vi "Find host address.vi"(0 "System number":i32=1 min=1 step=1, 1 "Port":i32=50000, 2 "Controller names":string[](array[string]), 3 "Mode":T1(ring), 5 "error in":errorcluster, 12 "Stop refnum":refnum<vi>) -> (14 "Address":string[](array[string]), 15 "ID":string[](array[string]), 16 "All Addresses":string[](array[string]), 17 "All IDs":string[](array[string]), 19 "error out":errorcluster)   [LabVIEW 2020]
doc: "Performs an UDP broadcast and returns IP addresses of all controllers matching Controller name. VI will also stop if Stop refnum or Local stop is TRUE.\n\nC-413: Controller names = C-413, Mode = Find XPort by UDP, Port = 30718\nC-413: Controller names = C-413, Mode = Find USR-K3 by UDP, Port = 1901\nC-702: Controller names = C-702, Mode = Find controller by UDP, Port = 50000\nC-867: Controller names = C-867, Mode = Find controller by UDP, Port = 50000\nC-884: Controller names = C-884, Mode = Find controller by UDP, Port = 50000\nC-885: Controller names = C-885, Mode = Find controller by UDP, Port = 50000\nC-886: Controller names = C-886, Mode = Find controller by UDP, Port = 50000\nC-891: Controller names = C-891, Mode = Find XPort by UDP, Port = 30718\nE-135: Controller names = E-135, Mode = Find USR-K3 by UDP, Port = 1901\nE-517: Controller names = E-517, Mode = Find controller by UDP, Port = 50000\nE-518: Controller names = E-518, Mode = Find controller by UDP, Port = 50000\nE-712: Controller names = E-712, Mode = Find controller by UDP, Port = 50000\nE-725: Controller names = E-725, Mode = Find XPort by UDP, Port = 30718\nE-727: Controller names = E-727, Mode = Find controller by UDP, Port = 50000\nE-753: Controller names = E-753, Mode = Find controller by UDP, Port = 50000\nE-754: Controller names = E-754, Mode = Find controller by UDP, Port = 50000\nE-871: Controller names = E-871, Mode = Find XPort by UDP, Port = 30718\nE-872: Controller names = E-872, Mode = Find controller by UDP, Port = 50000\nE-873: Controller names = E-873, Mode = Find XPort by UDP, Port = 30718\nE-874: Controller names = E-874, Mode = Find USR-K3 by UDP, Port = 1901\nF-206: Controller names = F-206, F-HEX, Mode = Find XPort by UDP, Port = 30718\nC-887, M-8X0: Controller names = M-8X0, HEXAPOD, Mode = Find XPort by UDP, Port = 30718"
uses:
  ProgramData/PI/LabVIEW/Low Level/Communication.llb/Available interfaces.ctl
  ProgramData/PI/LabVIEW/Low Level/Communication.llb/Global1.vi
  <vilib>/regexp/Match Regular Expression.xnode
panel:
  in  "stop":bool
  # "Performs an UDP broadcast and returns IP addresses of all controllers matching \"Controller name\"."
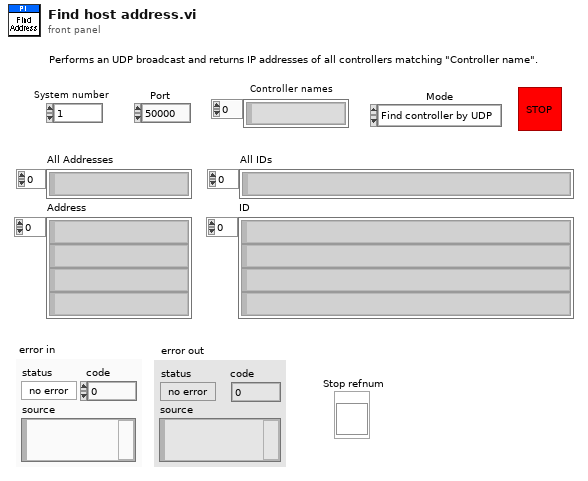
[diagram p1: front panel]
types:
  T1 = enum16{"Find controller by UDP", "Find XPort by UDP", "Find USR-K3 by UDP"}
  T2 = cluster{"Host address/name":string, "Port":i32, "Board":i32}
  T3 = typedef "Available interfaces.ctl" = u16
  T4 = cluster{"RS232 Portnumber":i32, "Timeout":i32, "RS232 Baud rate":u32, "Interface":T3, "GPIB Bus":i32, "GPIB Address":i32, "GPIB Mode":i32}
  T5 = cluster{"second":i32, "minute":i32, "hour":i32, "day of month":i32, "month":i32, "year":i32, "day of week":i32, "day of year":i32, "is DST":i32}
  T6 = cluster{"[0]":u8, "[1]":u8, "[2]":u8, "[3]":u8, "[4]":u8, "[5]":u8, "[6]":u8, "[7]":u8, "[8]":u8, "[9]":u8, "[10]":u8, "[11]":u8, "[12]":u8, "[13]":u8, "[14]":u8, "[15]":u8, "[16]":u8, "[17]":u8, "[18]":u8, "[19]":u8, "[20]":u8, "[21]":u8, "[22]":u8, "[23]":u8, "[24]":u8, "[25]":u8, "[26]":u8, "[27]":u8, "[28]":u8, "[29]":u8, "[30]":u8, "[31]":u8, "[32]":u8, "[33]":u8, "[34]":u8, "[35]":u8, "[36]":u8, "[37]":u8, "[38]":u8, "[39]":u8, "[40]":u8, "[41]":u8, "[42]":u8, "[43]":u8, "[44]":u8, "[45]":u8, "[46]":u8, "[47]":u8, "[48]":u8, "[49]":u8, "[50]":u8, "[51]":u8, "[52]":u8, "[53]":u8, "[54]":u8, "[55]":u8, "[56]":u8, "[57]":u8, "[58]":u8, "[59]":u8, "[60]":u8, "[61]":u8, "[62]":u8, "[63]":u8, "[64]":u8, "[65]":u8, "[66]":u8, "[67]":u8, "[68]":u8, "[69]":u8, "[70]":u8, "[71]":u8, "[72]":u8, "[73]":u8, "[74]":u8, "[75]":u8, "[76]":u8, "[77]":u8, "[78]":u8, "[79]":u8, "[80]":u8, "[81]":u8, "[82]":u8, "[83]":u8, "[84]":u8, "[85]":u8, "[86]":u8, "[87]":u8, "[88]":u8, "[89]":u8, "[90]":u8, "[91]":u8, "[92]":u8, "[93]":u8, "[94]":u8, "[95]":u8, "[96]":u8, "[97]":u8, "[98]":u8, "[99]":u8, "[100]":u8, "[101]":u8, "[102]":u8, "[103]":u8, "[104]":u8, "[105]":u8, "[106]":u8, "[107]":u8, "[108]":u8, "[109]":u8, "[110]":u8, "[111]":u8, "[112]":u8, "[113]":u8, "[114]":u8, "[115]":u8, "[116]":u8, "[117]":u8, "[118]":u8, "[119]":u8, "[120]":u8, "[121]":u8, "[122]":u8, "[123]":u8}
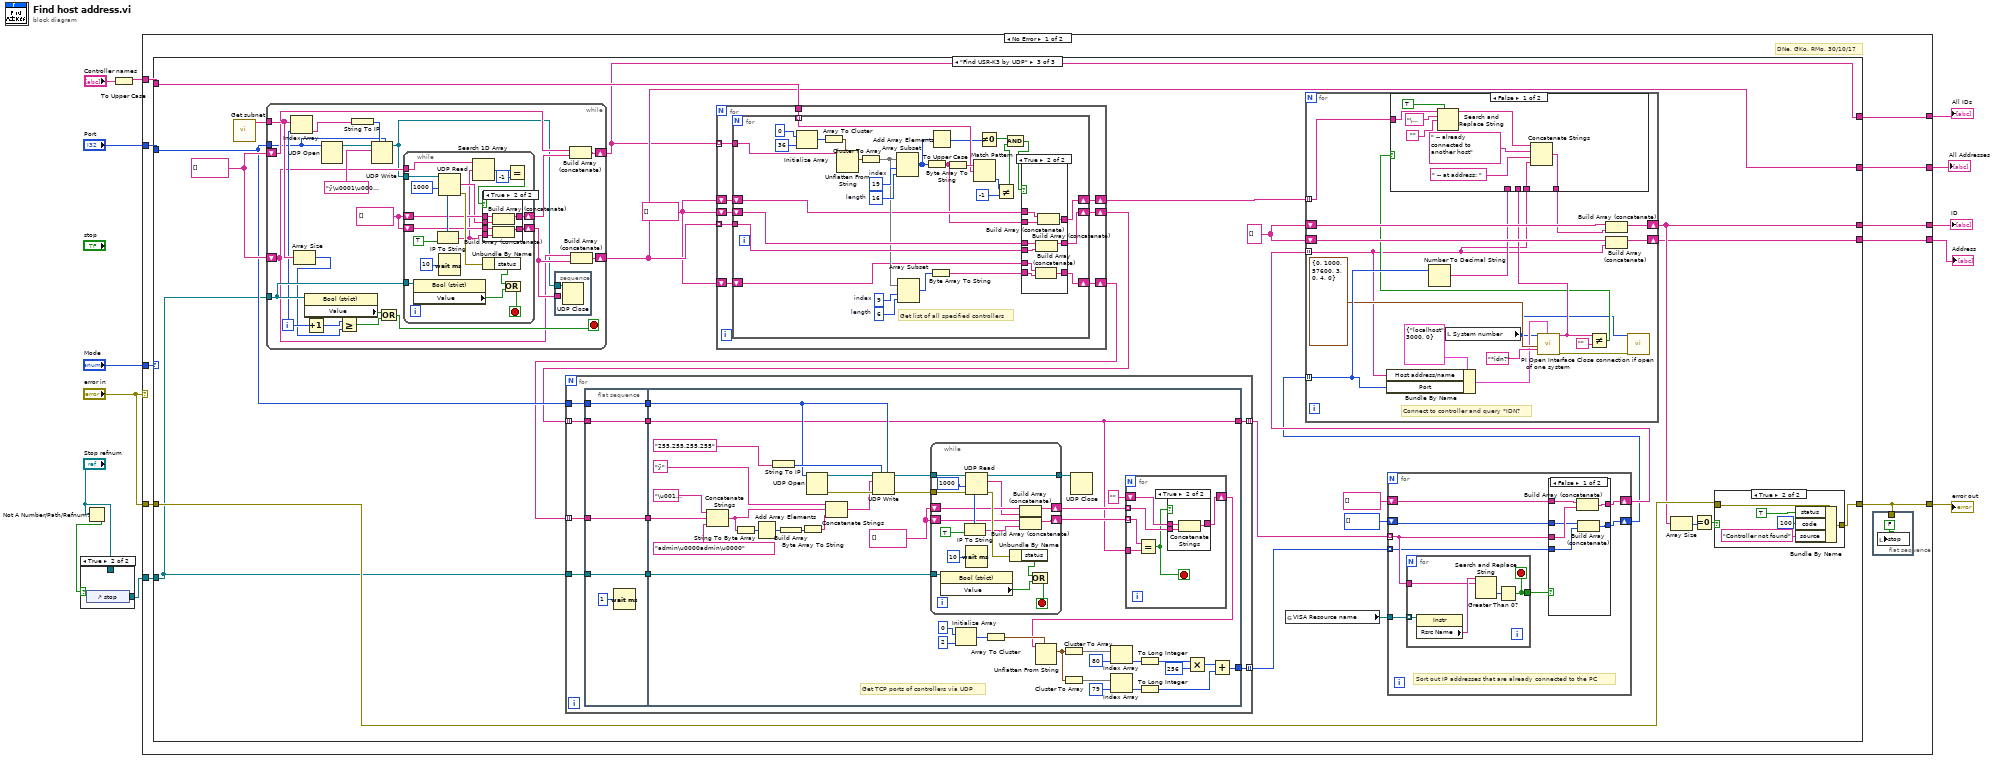
[diagram p0: block diagram]
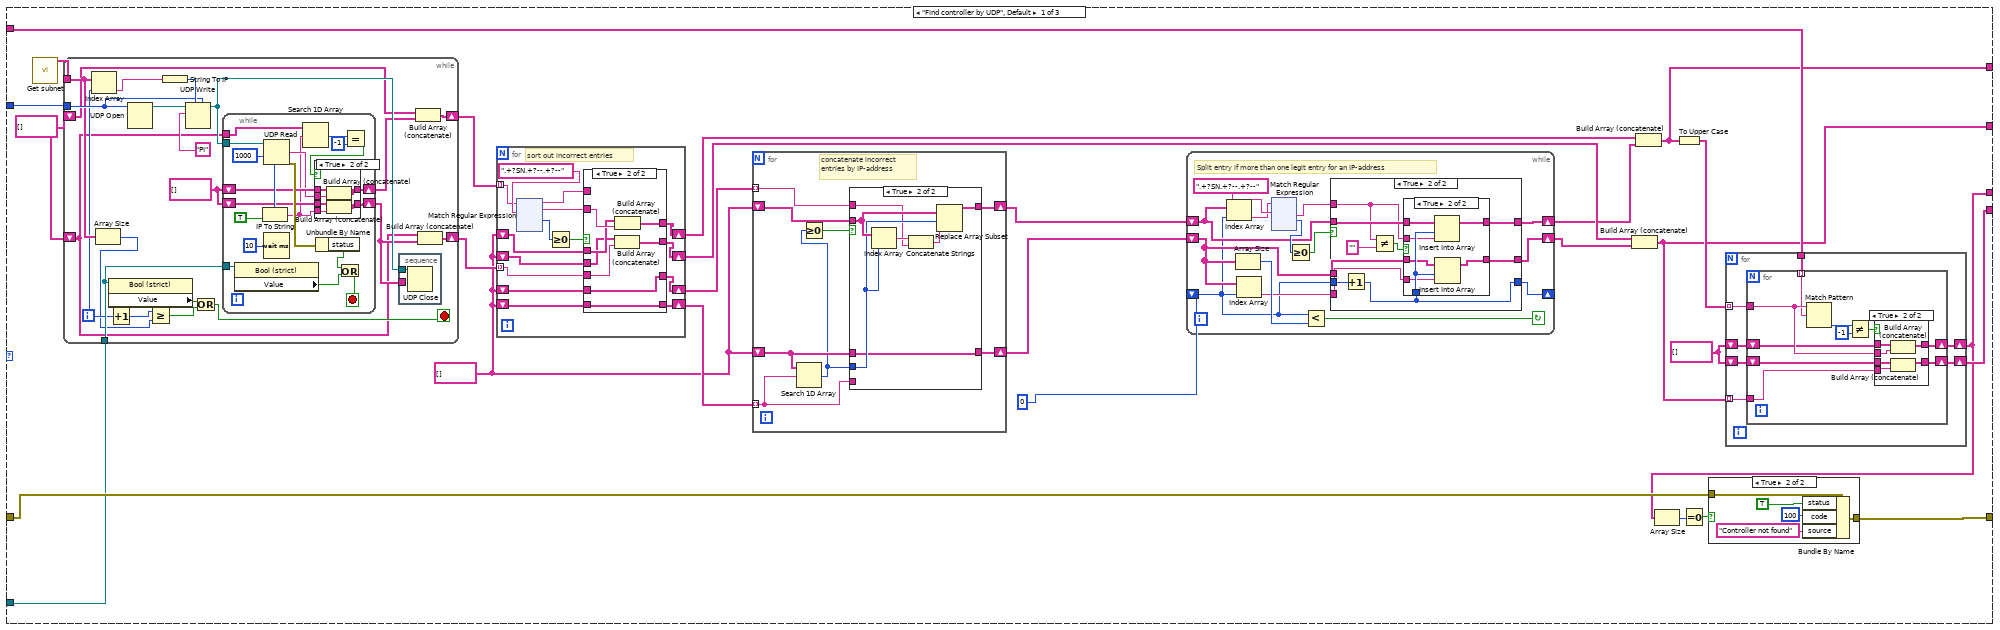
[diagram p3: hidden frame]
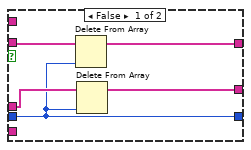
[diagram p4: hidden frame]
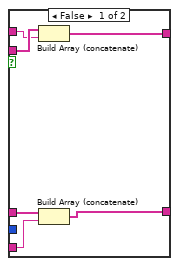
[diagram p6: hidden frame]
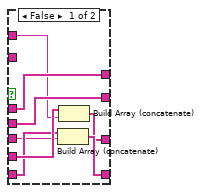
[diagram p7: hidden frame]
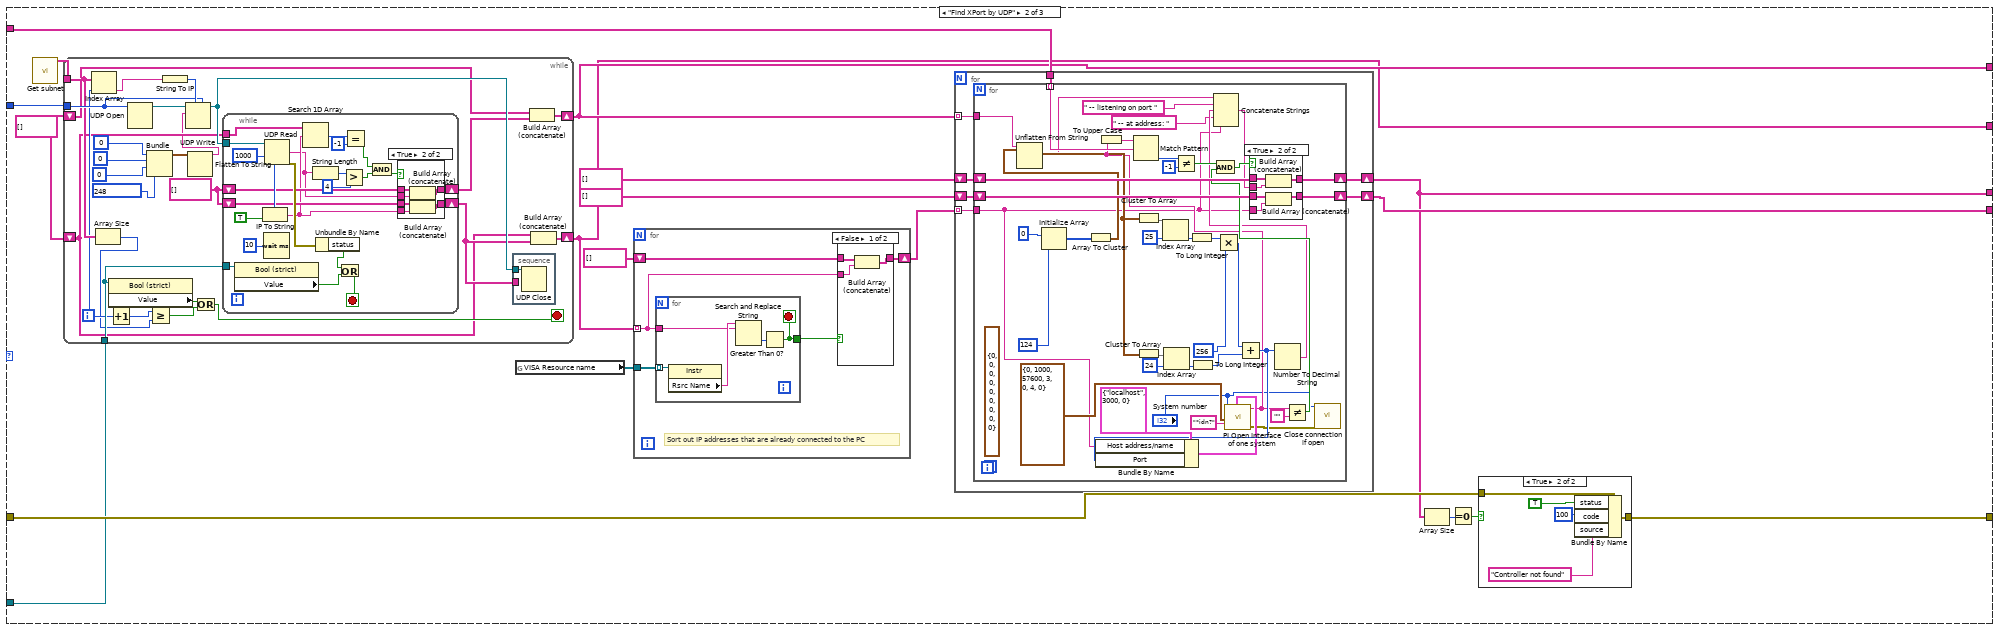
[diagram p11: hidden frame]
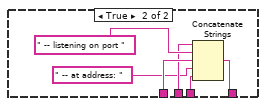
[diagram p17: hidden frame]
diagram:
  n1 = Not A Number/Path/Refnum?(number/path/refnum="Stop refnum") -> (NaN/Path/Refnum?=w7:bool)
  n2 = case shown="True" w7 {
    tunnel: [w14 w15] -> w5
    tunnel: "Stop refnum" -> [w14 _]
    frame False {
    }
    frame True {
      n3 = control-ref of="stop"() -> (w15:refnum<vi>)
    }
  }
  n4 = To Upper Case(1:"Controller names") -> (0:w4:string[])
  n5 = case shown="No Error" "error in" {
    tunnel: [w19 w880] -> w13
    tunnel: "error in" -> [w25 w880]
    tunnel: "Port" -> [w24 _]
    tunnel: "Mode" -> [w23 _]
    tunnel: w4 -> [w22 _]
    tunnel: [w21 string[] []] -> w2
    tunnel: [w17 string[] []] -> w9
    tunnel: [w18 string[] []] -> w8
    tunnel: w5 -> [w20 _]
    tunnel: [w16 string[] []] -> w1
    frame No Error {
      # "DNe, GKo, RMo, 30/10/17"
      n6 = case shown="\"Find USR-K3 by UDP\"" w23 {
        tunnel: w25 -> [w51 w466 w628]
        tunnel: [w50 w465 w627] -> w19
        tunnel: w24 -> [w49 w464 w621]
        tunnel: w22 -> [w40 w463 w626]
        tunnel: [w39 w457 w622] -> w21
        tunnel: [w48 w462 w617] -> w17
        tunnel: [w46 w460 w618] -> w18
        tunnel: w20 -> [w47 w461 w613]
        tunnel: [w36 w455 w623] -> w16
        frame "Find controller by UDP", Default {
          w28 = string[] []
          w44 = string[] []
          w27 = string[] []
          n7 = call "Get subnet.vi"() -> ("Subnet"=w45:string[])  [unwired: 19 out]
          n8 = while {
            tunnel: w49 -> [w389]
            tunnel: w47 -> [w386]
            tunnel: w45 -> [w387]
            shift-right: [w384] -> w41
            shift-left: w44 -> [w376]
            shift-right: [w378] -> w42
            shift-left: w44 -> [w372]
            i -> [w383]
            stop <- w380 stop-if-true
            w373 = string[] []
            n9 = Index Array(array=w387, index=w383) -> (element=w388:string)
            n10 = Array Size(array=w387) -> (size(s)=w379:i32)
            n11 = property class="Bool (strict)"(reference=w386) -> ("Value"=w385:bool)  [unwired: 1 in, 2 out]
            n12 = Increment(x=w383) -> (x+1=w382:i32)
            n13 = UDP Open(11:w389) -> (port=w392:refnum<k16>)  [unwired: 1 in, 5 out]
            n14 = Greater Or Equal?(x=w382, y=w379) -> (x >= y?=w381:bool)
            n15 = String To IP(1:w388) -> (0:w391:u32)
            n16 = UDP Write(address=w391, port or service name=w389, connection ID=w392, data in="PI") -> (3:w377:refnum<k16>)  [unwired: 1 in, 2 out]
            n17 = Or(x=w385, y=w381) -> (x .or. y?=w380:bool)
            n18 = while {
              tunnel: w377 -> [w413]
              tunnel: w386 -> [w409]
              shift-right: [w399] -> w375
              shift-left: w373 -> [w401]
              shift-right: [w397] -> w374
              shift-left: w373 -> [w398]
              tunnel: w372 -> [w395]
              stop <- w405 stop-if-true
              n19 = property class="Bool (strict)"(reference=w409) -> ("Value"=w408:bool)  [unwired: 1 in, 2 out]
              n20 = UDP Read(connection ID=w413, timeout ms (25000)=1000) -> (data out=w400:string, error out=w407:errorcluster, 6:w412:u32)  [unwired: 1 in, 3 out]
              n21 = IP To String(1:TRUE ("dot notation? (F)"), 2:w412) -> (0:w396:string)
              n22 = Wait (ms)(milliseconds to wait=u32 10) -> ()  [unwired: 1 out]
              n23 = Search 1D Array(1D array=w395, element=w396) -> (index of element=w404:i32)  [unwired: 1 out]
              n24 = Unbundle By Name(w407) -> ("status"=w406:bool)
              n25 = Or(x=w406, y=w408) -> (x .or. y?=w405:bool)
              n26 = Equal?(x=w404, y=-1) -> (x = y?=w402:bool)
              n27 = case shown="True" w402 {
                tunnel: w401 -> [w415 w421]
                tunnel: w400 -> [_ w416]
                tunnel: [w415 w420] -> w399
                tunnel: w398 -> [w414 w419]
                tunnel: [w414 w418] -> w397
                tunnel: w396 -> [_ w417]
                frame False {
                }
                frame True {
                  n28 = Build Array (concatenate)(w421, w416) -> (w420:string[])
                  n29 = Build Array (concatenate)(w419, w417) -> (w418:string[])
                }
              }
            }
            n30 = stacked-sequence {
              tunnel: w377 -> [w393]
              tunnel: w374 -> [_]
              frame #0 {
                n31 = UDP Close(connection ID=w393) -> ()  [unwired: 1 in, 2 out]
              }
            }
            n32 = Build Array (concatenate)(w376, w375) -> (w384:string[])
            n33 = Build Array (concatenate)(w372, w374) -> (w378:string[])
          }
          n34 = for {
            tunnel: w41 -> [w240] mode=indexing
            tunnel: w42 -> [w236] mode=indexing
            shift-right: [w237] -> w38
            shift-left: w28 -> [w238]
            shift-right: [w234] -> w37
            shift-left: w28 -> [w235]
            shift-right: [w229] -> w34
            shift-left: w28 -> [w230]
            shift-right: [w227] -> w35
            shift-left: w28 -> [w231]
            # "sort out incorrect entries"
            n35 = xnode "Match Regular Expression"("input string"=w240, "regular expression"=".+?SN.+?--.+?--") -> ("before match"=w228:string, "whole match"=w239:string, "offset past match"=w233:i32)  [unwired: 2 in, 4 out]
            n36 = Greater Or Equal To 0?(x=w233) -> (x >= 0?=w232:bool)
            n37 = case shown="True" w232 {
              tunnel: w239 -> [_ w257]
              tunnel: w238 -> [w248 w256]
              tunnel: [w248 w255] -> w237
              tunnel: w236 -> [w245 w254]
              tunnel: w235 -> [w249 w253]
              tunnel: [w249 w252] -> w234
              tunnel: w231 -> [w247 w250]
              tunnel: w230 -> [w246 w251]
              tunnel: [w244 w251] -> w229
              tunnel: w228 -> [w243 _]
              tunnel: [w242 w250] -> w227
              frame False {
                n38 = Build Array (concatenate)(w246, w245) -> (w244:string[])
                n39 = Build Array (concatenate)(w247, w243) -> (w242:string[])
              }
              frame True {
                n40 = Build Array (concatenate)(w253, w254) -> (w252:string[])
                n41 = Build Array (concatenate)(w256, w257) -> (w255:string[])
              }
            }
          }
          n42 = for {
            tunnel: w35 -> [w210] mode=indexing
            tunnel: w34 -> [w209] mode=indexing
            shift-right: [w212] -> w33
            shift-left: w28 -> [w213]
            shift-right: [w211] -> w32
            shift-left: w28 -> [w208]
            # "concatenate incorrect\nentries by IP-address"
            n43 = Search 1D Array(1D array=w208, element=w209) -> (index of element=w206:i32)  [unwired: 1 out]
            n44 = Greater Or Equal To 0?(x=w206) -> (x >= 0?=w207:bool)
            n45 = case shown="True" w207 {
              tunnel: w213 -> [w219 w226]
              tunnel: w208 -> [w218 w220]
              tunnel: [w217 w221] -> w212
              tunnel: [w216 w220] -> w211
              tunnel: w210 -> [w215 w223]
              tunnel: w209 -> [w214 _]
              tunnel: w206 -> [_ w225]
              frame False {
                n46 = Build Array (concatenate)(w219, w215) -> (w217:string[])
                n47 = Build Array (concatenate)(w218, w214) -> (w216:string[])
              }
              frame True {
                n48 = Index Array(array=w226, index=w225) -> (element=w224:string)
                n49 = Concatenate Strings(w224, w223) -> (w222:string)
                n50 = Replace Array Subset(array=w226, new element=w222, index=w225) -> (w221:string[])
              }
            }
          }
          n51 = while {
            shift-right: [w61] -> w30
            shift-left: w33 -> [w59]
            shift-right: [w60] -> w31
            shift-left: w32 -> [w58]
            shift-right: [w54] -> _
            shift-left: 0 -> [w55]
            stop <- w67 continue-if-true
            # "Split entry if more than one legit entry for an IP-address"
            n52 = Index Array(array=w59, index=w55) -> (element=w65:string)
            n53 = Array Size(array=w58) -> (size(s)=w62:i32)
            n54 = Index Array(array=w58, index=w55) -> (element=w57:string)
            n55 = xnode "Match Regular Expression"("input string"=w65, "regular expression"=".+?SN.+?--.+?--") -> ("after match"=w56:string, "offset past match"=w64:i32)  [unwired: 2 in, 5 out]
            n56 = Greater Or Equal To 0?(x=w64) -> (x >= 0?=w63:bool)
            n57 = Less?(x=w55, y=w62) -> (x < y?=w67:bool)
            n58 = case shown="True" w63 {
              tunnel: w58 -> [w71 w81]
              tunnel: w55 -> [w68 w82]
              tunnel: [w69 w77] -> w61
              tunnel: [w72 w80] -> w60
              tunnel: w59 -> [w70 w79]
              tunnel: w56 -> [_ w75]
              tunnel: w57 -> [_ w78]
              tunnel: [w68 w73] -> w54
              frame False {
                n59 = Delete From Array(array=w70, index=w68) -> (array with subset deleted=w69:string[])  [unwired: 1 in, 1 out]
                n60 = Delete From Array(array=w71, index=w68) -> (array with subset deleted=w72:string[])  [unwired: 1 in, 1 out]
              }
              frame True {
                n61 = Increment(x=w82) -> (x+1=w73:i32)
                n62 = Not Equal?(x=w75, y="") -> (x != y?=w76:bool)
                n63 = case shown="True" w76 {
                  tunnel: w73 -> [_ w91]
                  tunnel: w81 -> [w83 w90]
                  tunnel: [w83 w89] -> w80
                  tunnel: w79 -> [w84 w88]
                  tunnel: w75 -> [_ w87]
                  tunnel: w78 -> [_ w86]
                  tunnel: [w84 w85] -> w77
                  frame False {
                  }
                  frame True {
                    n64 = Insert Into Array(array=w88, index=w91, new element=w87) -> (w85:string[])
                    n65 = Insert Into Array(array=w90, index=w91, new element=w86) -> (w89:string[])
                  }
                }
              }
            }
          }
          n66 = Build Array (concatenate)(w37, w31) -> (w36:string[])
          n67 = Build Array (concatenate)(w38, w30) -> (w39:string[])
          n68 = To Upper Case(1:w39) -> (0:w43:string[])
          n69 = for {
            tunnel: w43 -> [w428] mode=indexing
            shift-right: [w427] -> w46
            shift-left: w27 -> [w424]
            shift-right: [w425] -> w48
            shift-left: w27 -> [w426]
            tunnel: w40 -> [w423]
            tunnel: w36 -> [w422] mode=indexing
            n70 = for {
              tunnel: w428 -> [w435]
              tunnel: w423 -> [w430] mode=indexing
              shift-right: [w434] -> w427
              shift-left: w424 -> [w431]
              shift-right: [w432] -> w425
              shift-left: w426 -> [w433]
              tunnel: w422 -> [w429]
              n71 = Match Pattern(string=w435, regular expression=w430) -> (offset past match=w438:i32)  [unwired: 4 out]
              n72 = Not Equal?(x=w438, y=-1) -> (x != y?=w436:bool)
              n73 = case shown="True" w436 {
                tunnel: w435 -> [_ w442]
                tunnel: [w440 w444] -> w434
                tunnel: w433 -> [w439 w446]
                tunnel: [w439 w445] -> w432
                tunnel: w431 -> [w440 w443]
                tunnel: w429 -> [_ w441]
                frame False {
                }
                frame True {
                  n74 = Build Array (concatenate)(w443, w442) -> (w444:string[])
                  n75 = Build Array (concatenate)(w446, w441) -> (w445:string[])
                }
              }
            }
          }
          n76 = Array Size(array=w46) -> (size(s)=w53:i32)
          n77 = Equal To 0?(x=w53) -> (x = 0?=w52:bool)
          n78 = case shown="True" w52 {
            tunnel: [w447 w449] -> w50
            tunnel: w51 -> [w447 w448]
            frame False {
            }
            frame True {
              n79 = Bundle By Name(cluster=w448, "status"=TRUE, "code"=100 ("Bundle Element"), "source"="Controller not found" ("Bundle Element")) -> (w449:errorcluster)
            }
          }
        }
        frame "Find XPort by UDP" {
          w458 = string[] []
          n80 = call "Get subnet.vi"() -> ("Subnet"=w459:string[])  [unwired: 19 out]
          n81 = while {
            tunnel: w464 -> [w508]
            tunnel: w461 -> [w505]
            tunnel: w459 -> [w506]
            shift-right: [w503] -> w457
            shift-left: w458 -> [w495]
            shift-right: [w497] -> w455
            shift-left: w458 -> [w491]
            i -> [w502]
            stop <- w499 stop-if-true
            w492 = string[] []
            n82 = Index Array(array=w506, index=w502) -> (element=w507:string)
            n83 = Array Size(array=w506) -> (size(s)=w498:i32)
            n84 = property class="Bool (strict)"(reference=w505) -> ("Value"=w504:bool)  [unwired: 1 in, 2 out]
            n85 = Increment(x=w502) -> (x+1=w501:i32)
            n86 = UDP Open(11:w508) -> (port=w510:refnum<k16>)  [unwired: 1 in, 5 out]
            n87 = Bundle(u8 0, u8 0, u8 0, u8 248) -> (w490:cluster{u8, u8, u8, u8})  [unwired: 1 out]
            n88 = Greater Or Equal?(x=w501, y=w498) -> (x >= y?=w500:bool)
            n89 = String To IP(1:w507) -> (0:w509:u32)
            n90 = Flatten To String(anything=w490) -> (data string=w485:string)  [unwired: 1 in, 4 out]
            n91 = UDP Write(address=w509, port or service name=w508, connection ID=w510, data in=w485) -> (3:w496:refnum<k16>)  [unwired: 1 in, 2 out]
            n92 = Or(x=w504, y=w500) -> (x .or. y?=w499:bool)
            n93 = while {
              tunnel: w496 -> [w535]
              tunnel: w505 -> [w531]
              shift-right: [w523] -> w494
              shift-left: w492 -> [w524]
              shift-right: [w521] -> w493
              shift-left: w492 -> [w522]
              tunnel: w491 -> [w519]
              stop <- w527 stop-if-true
              n94 = property class="Bool (strict)"(reference=w531) -> ("Value"=w530:bool)  [unwired: 1 in, 2 out]
              n95 = Wait (ms)(milliseconds to wait=u32 10) -> ()  [unwired: 1 out]
              n96 = UDP Read(connection ID=w535, timeout ms (25000)=1000) -> (data out=w518:string, error out=w529:errorcluster, 6:w534:u32)  [unwired: 1 in, 3 out]
              n97 = IP To String(1:TRUE ("dot notation? (F)"), 2:w534) -> (0:w520:string)
              n98 = Search 1D Array(1D array=w519, element=w520) -> (index of element=w526:i32)  [unwired: 1 out]
              n99 = String Length(string=w518) -> (length=w517:i32)
              n100 = Unbundle By Name(w529) -> ("status"=w528:bool)
              n101 = Or(x=w528, y=w530) -> (x .or. y?=w527:bool)
              n102 = Greater?(x=w517, y=4) -> (0:w515:bool)
              n103 = Equal?(x=w526, y=-1) -> (x = y?=w514:bool)
              n104 = And(x=w514, y=w515) -> (x .and. y?=w513:bool)
              n105 = case shown="True" w513 {
                tunnel: w524 -> [w537 w543]
                tunnel: w518 -> [_ w538]
                tunnel: [w537 w542] -> w523
                tunnel: w522 -> [w536 w541]
                tunnel: [w536 w540] -> w521
                tunnel: w520 -> [_ w539]
                frame False {
                }
                frame True {
                  n106 = Build Array (concatenate)(w543, w538) -> (w542:string[])
                  n107 = Build Array (concatenate)(w541, w539) -> (w540:string[])
                }
              }
            }
            n108 = stacked-sequence {
              tunnel: w496 -> [w511]
              tunnel: w493 -> [_]
              frame #0 {
                n109 = UDP Close(connection ID=w511) -> ()  [unwired: 1 in, 2 out]
              }
            }
            n110 = Build Array (concatenate)(w495, w494) -> (w503:string[])
            n111 = Build Array (concatenate)(w491, w493) -> (w497:string[])
          }
          n112 = global read "Global1.vi" "VISA Resource name"() -> (w456:refnum<visa-resource-name>[])
          n113 = for {
            tunnel: w456 -> [w473]
            shift-right: [w471] -> w453
            shift-left: string[] [] -> [w474]
            tunnel: w455 -> [w472] mode=indexing
            # "Sort out IP addresses that are already connected to the PC"
            n114 = for {
              tunnel: w472 -> [w481]
              tunnel: [w484] -> w475
              tunnel: w473 -> [w483] mode=indexing
              stop <- w484 stop-if-true
              n115 = property class="Instr"(reference=w483) -> ("Rsrc Name"=w482:string)  [unwired: 1 in, 2 out]
              n116 = Search and Replace String(input string=w482, search string=w481) -> (offset past replacement=w480:i32)  [unwired: 1 in, 8 out]
              n117 = Greater Than 0?(x=w480) -> (x > 0?=w484:bool)
            }
            n118 = case shown="False" w475 {
              tunnel: w474 -> [w478 w479]
              tunnel: w472 -> [w477 _]
              tunnel: [w476 w479] -> w471
              frame False {
                n119 = Build Array (concatenate)(w478, w477) -> (w476:string[])
              }
              frame True {
              }
            }
          }
          n120 = for {
            shift-right: [w550] -> w460
            shift-left: string[] [] -> [w547]
            shift-right: [w548] -> w462
            shift-left: string[] [] -> [w549]
            tunnel: w463 -> [w546]
            tunnel: w453 -> [w545] mode=indexing
            tunnel: w457 -> [w544] mode=indexing
            n121 = for {
              tunnel: w546 -> [w585] mode=indexing
              shift-right: [w589] -> w550
              shift-left: w547 -> [w586]
              shift-right: [w587] -> w548
              shift-left: w549 -> [w588]
              tunnel: w545 -> [w553]
              tunnel: w544 -> [w555]
              (unwired) T5 {"second"=0, "minute"=0, "hour"=0, "day of month"=0, "month"=0, "year"=0, "day of week"=0, "day of year"=0, "is DST"=0} ("type")
              n122 = Initialize Array(u8 0 ("element"), 124 ("dimension size")) -> (w584:u8[])
              n123 = Array To Cluster(array=w584) -> (cluster=w571:T6)
              n124 = Unflatten From String(type=w571, binary string=w555) -> (value=w570:T6)  [unwired: 1 in, 4 out]
              n125 = Cluster To Array(cluster=w570) -> (array=w581:u8[])
              n126 = Cluster To Array(cluster=w570) -> (array=w574:u8[])
              n127 = Index Array(array=w581, index=25) -> (element=w579:u8)
              n128 = Index Array(array=w574, index=24) -> (element=w576:u8)
              n129 = To Long Integer(number=w579) -> (32bit integer=w578:i32)
              n130 = To Long Integer(number=w576) -> (32bit integer=w573:i32)
              n131 = Multiply(x=w578, y=256) -> (x*y=w572:i32)
              n132 = Add(x=w572, y=w573) -> (x+y=w566:i32)
              n133 = Bundle By Name(cluster=T2 {"Host address/name"="localhost", "Port"=3000, "Board"=0} ("TCP/IP\nConfiguration"), "Host address/name"=w553, "Port"=w566) -> (w565:T2)
              n134 = call "PI Open Interface of one system.vi"("System number"="System number", "Interface configuration"=T4 {"RS232 Portnumber"=0, "Timeout"=1000, "RS232 Baud rate"=57600, "Interface"=3, "GPIB Bus"=0, "GPIB Address"=4, "GPIB Mode"=0}, "String to Send"="*idn?", "TCP/IP\nConfiguration"=w565) -> ("String read"=w556:string, "error out"=w551:errorcluster)  [unwired: 8 in, 6 out]
              n135 = To Upper Case(1:w556) -> (0:w557:string)
              n136 = Match Pattern(string=w557, regular expression=w585) -> (offset past match=w591:i32)  [unwired: 4 out]
              n137 = Not Equal?(x=w591, y=-1) -> (x != y?=w563:bool)
              n138 = Number To Decimal String(number=w566) -> (decimal integer string=w558:string)  [unwired: 1 out]
              n139 = Concatenate Strings(w556, " -- listening on port " ("string"), w558, " -- at address: " ("string"), w553) -> (w560:string)
              n140 = Not Equal?(x=w556, y="") -> (x != y?=w561:bool)
              n141 = And(x=w563, y=w561) -> (x .and. y?=w562:bool)
              n142 = case shown="True" w562 {
                tunnel: w560 -> [_ w595]
                tunnel: [w593 w597] -> w589
                tunnel: w588 -> [w592 w599]
                tunnel: [w592 w598] -> w587
                tunnel: w586 -> [w593 w596]
                tunnel: w553 -> [_ w594]
                frame False {
                }
                frame True {
                  n143 = Build Array (concatenate)(w596, w595) -> (w597:string[])
                  n144 = Build Array (concatenate)(w599, w594) -> (w598:string[])
                }
              }
              n145 = call "Close connection if open.vi"("System no."="System number", "error in"=w551) -> ()  [unwired: 1 in, 17 out]
            }
          }
          n146 = Array Size(array=w460) -> (size(s)=w468:i32)
          n147 = Equal To 0?(x=w468) -> (x = 0?=w467:bool)
          n148 = case shown="True" w467 {
            tunnel: [w600 w602] -> w465
            tunnel: w466 -> [w600 w601]
            frame False {
            }
            frame True {
              n149 = Bundle By Name(cluster=w601, "status"=TRUE, "code"=100 ("Bundle Element"), "source"="Controller not found" ("Bundle Element")) -> (w602:errorcluster)
            }
          }
        }
        frame "Find USR-K3 by UDP" {
          w619 = string[] []
          w615 = string[] []
          w625 = string[] []
          n150 = call "Get subnet.vi"() -> ("Subnet"=w624:string[])  [unwired: 19 out]
          n151 = while {
            tunnel: w613 -> [w835]
            tunnel: w624 -> [w836]
            shift-right: [w833] -> w622
            shift-left: w625 -> [w826]
            shift-right: [w827] -> w623
            shift-left: w625 -> [w822]
            tunnel: w621 -> [w821]
            i -> [w832]
            stop <- w829 stop-if-true
            w823 = string[] []
            n152 = Index Array(array=w836, index=w832) -> (element=w837:string)
            n153 = Array Size(array=w836) -> (size(s)=w828:i32)
            n154 = property class="Bool (strict)"(reference=w835) -> ("Value"=w834:bool)  [unwired: 1 in, 2 out]
            n155 = Increment(x=w832) -> (x+1=w831:i32)
            n156 = UDP Open(11:w821) -> (port=w840:refnum<k16>)  [unwired: 1 in, 5 out]
            n157 = Greater Or Equal?(x=w831, y=w828) -> (x >= y?=w830:bool)
            n158 = String To IP(1:w837) -> (0:w839:u32)
            n159 = UDP Write(address=w839, port or service name=w821, connection ID=w840, data in="ÿ\u0001\u0001\u0002") -> (3:w820:refnum<k16>)  [unwired: 1 in, 2 out]
            n160 = Or(x=w834, y=w830) -> (x .or. y?=w829:bool)
            n161 = while {
              tunnel: w820 -> [w861]
              tunnel: w835 -> [w857]
              shift-right: [w847] -> w825
              shift-left: w823 -> [w849]
              shift-right: [w845] -> w824
              shift-left: w823 -> [w846]
              tunnel: w822 -> [w843]
              stop <- w853 stop-if-true
              n162 = property class="Bool (strict)"(reference=w857) -> ("Value"=w856:bool)  [unwired: 1 in, 2 out]
              n163 = UDP Read(connection ID=w861, timeout ms (25000)=1000) -> (data out=w848:string, error out=w855:errorcluster, 6:w860:u32)  [unwired: 1 in, 3 out]
              n164 = IP To String(1:TRUE ("dot notation? (F)"), 2:w860) -> (0:w844:string)
              n165 = Wait (ms)(milliseconds to wait=u32 10) -> ()  [unwired: 1 out]
              n166 = Search 1D Array(1D array=w843, element=w844) -> (index of element=w852:i32)  [unwired: 1 out]
              n167 = Unbundle By Name(w855) -> ("status"=w854:bool)
              n168 = Or(x=w854, y=w856) -> (x .or. y?=w853:bool)
              n169 = Equal?(x=w852, y=-1) -> (x = y?=w850:bool)
              n170 = case shown="True" w850 {
                tunnel: w849 -> [w863 w869]
                tunnel: w848 -> [_ w864]
                tunnel: [w863 w868] -> w847
                tunnel: w846 -> [w862 w867]
                tunnel: [w862 w866] -> w845
                tunnel: w844 -> [_ w865]
                frame False {
                }
                frame True {
                  n171 = Build Array (concatenate)(w869, w864) -> (w868:string[])
                  n172 = Build Array (concatenate)(w867, w865) -> (w866:string[])
                }
              }
            }
            n173 = stacked-sequence {
              tunnel: w820 -> [w841]
              tunnel: w824 -> [_]
              frame #0 {
                n174 = UDP Close(connection ID=w841) -> ()  [unwired: 1 in, 2 out]
              }
            }
            n175 = Build Array (concatenate)(w826, w825) -> (w833:string[])
            n176 = Build Array (concatenate)(w822, w824) -> (w827:string[])
          }
          n177 = for {
            shift-right: [w776] -> w620
            shift-left: w615 -> [w777]
            tunnel: w626 -> [w775]
            tunnel: w623 -> [w774] mode=indexing
            tunnel: w622 -> [w773] mode=indexing
            shift-right: [w771] -> w616
            shift-left: w615 -> [w772]
            shift-right: [w769] -> w614
            shift-left: w615 -> [w770]
            n178 = for {
              tunnel: w775 -> [w798] mode=indexing
              shift-right: [w795] -> w776
              shift-left: w777 -> [w797]
              tunnel: w774 -> [w796]
              tunnel: w773 -> [w785]
              shift-right: [w790] -> w771
              shift-left: w772 -> [w789]
              shift-right: [w786] -> w769
              shift-left: w770 -> [w787]
              w794 = 6  # length
              w793 = 9  # index
              w806 = 16  # length
              w807 = 19  # index
              # "Get list of all specified controllers"
              n179 = Initialize Array(u8 0 ("element"), 36 ("dimension size")) -> (w803:u8[])
              n180 = Array To Cluster(array=w803) -> (cluster=w804:T6)
              n181 = Unflatten From String(type=w804, binary string=w785) -> (value=w805:T6)  [unwired: 1 in, 4 out]
              n182 = Cluster To Array(cluster=w805) -> (array=w792:u8[])
              n183 = Array Subset(array=w792, index=w807, length=w806) -> (w783:u8[])
              n184 = Array Subset(array=w792, index=w793, length=w794) -> (w791:u8[])
              n185 = Byte Array To String(unsigned byte array=w783) -> (string=w784:string)
              n186 = Byte Array To String(unsigned byte array=w791) -> (string=w788:string)
              n187 = Add Array Elements(numeric array=w783) -> (sum=w782:u8)
              n188 = To Upper Case(1:w784) -> (0:w800:string)
              n189 = Match Pattern(string=w800, regular expression=w798) -> (offset past match=w780:i32)  [unwired: 4 out]
              n190 = Not Equal To 0?(x=w782) -> (x != 0?=w781:bool)
              n191 = Not Equal?(x=w780, y=-1) -> (x != y?=w779:bool)
              n192 = And(x=w781, y=w779) -> (x .and. y?=w778:bool)
              n193 = case shown="True" w778 {
                tunnel: [w810 w819] -> w795
                tunnel: w797 -> [w810 w818]
                tunnel: w796 -> [_ w817]
                tunnel: [w809 w816] -> w790
                tunnel: w788 -> [_ w815]
                tunnel: w789 -> [w809 w814]
                tunnel: w787 -> [w808 w813]
                tunnel: [w808 w812] -> w786
                tunnel: w784 -> [_ w811]
                frame False {
                }
                frame True {
                  n194 = Build Array (concatenate)(w814, w815) -> (w816:string[])
                  n195 = Build Array (concatenate)(w818, w817) -> (w819:string[])
                  n196 = Build Array (concatenate)(w813, w811) -> (w812:string[])
                }
              }
            }
          }
          n197 = for {
            tunnel: w621 -> [w692]
            tunnel: w620 -> [w690] mode=indexing
            tunnel: [w689] -> w609 mode=indexing
            tunnel: [w694] -> w610 mode=indexing
            tunnel: w616 -> [w693] mode=indexing
            tunnel: w613 -> [w691]
            n198 = flat-sequence {
              tunnel: w690 -> [w696]
              tunnel: w691 -> [w697]
              tunnel: w692 -> [w698]
              tunnel: w693 -> [w699]
              tunnel: [w699] -> w688
              tunnel: [w698] -> w687
              tunnel: [w697] -> w686
              tunnel: [w696] -> w685
              tunnel: [w723] -> w694
              tunnel: [w700] -> w689
              tunnel: w688 -> [w721]
              tunnel: w687 -> [w712]
              tunnel: w686 -> [w710]
              tunnel: w685 -> [w700]
              frame #0 {
                n199 = Wait (ms)(milliseconds to wait=u32 1) -> ()  [unwired: 1 out]
              }
              frame #1 {
                w708 = string[] []
                # "Get TCP ports of controllers via UDP"
                n200 = Concatenate Strings("\u0013\u0003" ("data in"), w721, "admin\u0000admin\u0000" ("data in")) -> (w715:string)
                n201 = String To Byte Array(string=w715) -> (unsigned byte array=w718:u8[])
                n202 = Add Array Elements(numeric array=w718) -> (sum=w717:u8)
                n203 = String To IP(1:"255.255.255.255" ("name")) -> (0:w713:u32)
                n204 = Build Array(w717) -> (w716:u8[])
                n205 = Byte Array To String(unsigned byte array=w716) -> (string=w714:string)
                n206 = UDP Open(11:w712) -> (port=w739:refnum<k16>, 0:w740:errorcluster)  [unwired: 1 in, 4 out]
                n207 = Concatenate Strings("ÿ" ("data in"), w715, w714) -> (w711:string)
                n208 = UDP Write(address=w713, port or service name=w712, connection ID=w739, data in=w711, 8:w740) -> (error out=w701:errorcluster, 3:w709:refnum<k16>)  [unwired: 1 out]
                n209 = while {
                  tunnel: w709 -> [w768]
                  tunnel: w710 -> [w764]
                  shift-right: [w757] -> w706
                  shift-left: w708 -> [w759]
                  shift-right: [w755] -> w705
                  shift-left: w708 -> [w756]
                  tunnel: [w752] -> w704
                  tunnel: w701 -> [w751]
                  stop <- w760 stop-if-true
                  n210 = property class="Bool (strict)"(reference=w764) -> ("Value"=w763:bool)  [unwired: 1 in, 2 out]
                  n211 = UDP Read(connection ID=w768, timeout ms (25000)=1000, 8:w751) -> (data out=w758:string, error out=w762:errorcluster, 3:w752:refnum<k16>, 6:w767:u32)  [unwired: 2 out]
                  n212 = IP To String(1:TRUE ("dot notation? (F)"), 2:w767) -> (0:w754:string)
                  n213 = Wait (ms)(milliseconds to wait=u32 10) -> ()  [unwired: 1 out]
                  n214 = Unbundle By Name(w762) -> ("status"=w761:bool)
                  n215 = Build Array (concatenate)(w759, w758) -> (w757:string[])
                  n216 = Build Array (concatenate)(w756, w754) -> (w755:string[])
                  n217 = Or(x=w761, y=w763) -> (x .or. y?=w760:bool)
                }
                n218 = Initialize Array(u8 0 ("element"), 2 ("dimension size")) -> (w737:u8[])
                n219 = Array To Cluster(array=w737) -> (cluster=w738:T6)
                n220 = UDP Close(connection ID=w704) -> ()  [unwired: 1 in, 2 out]
                n221 = for {
                  shift-right: [w744] -> w703
                  shift-left: "" -> [w745]
                  tunnel: w706 -> [w743] mode=indexing
                  tunnel: w705 -> [w742] mode=indexing
                  tunnel: w700 -> [w746]
                  stop <- w741 stop-if-true
                  n222 = Equal?(x=w742, y=w746) -> (x = y?=w741:bool)
                  n223 = case shown="True" w741 {
                    tunnel: w745 -> [w747 w750]
                    tunnel: w743 -> [_ w749]
                    tunnel: [w747 w748] -> w744
                    frame False {
                    }
                    frame True {
                      n224 = Concatenate Strings(w750, w749) -> (w748:string)
                    }
                  }
                }
                n225 = Unflatten From String(type=w738, binary string=w703) -> (value=w725:T6)  [unwired: 1 in, 4 out]
                n226 = Cluster To Array(cluster=w725) -> (array=w724:u8[])
                n227 = Cluster To Array(cluster=w725) -> (array=w728:u8[])
                n228 = Index Array(array=w724, index=80) -> (element=w733:u8)
                n229 = Index Array(array=w728, index=79) -> (element=w730:u8)
                n230 = To Long Integer(number=w733) -> (32bit integer=w732:i32)
                n231 = To Long Integer(number=w730) -> (32bit integer=w727:i32)
                n232 = Multiply(x=w732, y=256) -> (x*y=w726:i32)
                n233 = Add(x=w726, y=w727) -> (x+y=w723:i32)
              }
            }
          }
          n234 = global read "Global1.vi" "VISA Resource name"() -> (w612:refnum<visa-resource-name>[])
          n235 = for {
            tunnel: w612 -> [w636]
            shift-right: [w634] -> w607
            shift-left: string[] [] -> [w637]
            tunnel: w609 -> [w635] mode=indexing
            tunnel: w610 -> [w633] mode=indexing
            shift-right: [w631] -> w606
            shift-left: i32[] [] -> [w632]
            # "Sort out IP addresses that are already connected to the PC"
            n236 = for {
              tunnel: w635 -> [w648]
              tunnel: [w651] -> w638
              tunnel: w636 -> [w650] mode=indexing
              stop <- w651 stop-if-true
              n237 = property class="Instr"(reference=w650) -> ("Rsrc Name"=w649:string)  [unwired: 1 in, 2 out]
              n238 = Search and Replace String(input string=w649, search string=w648) -> (offset past replacement=w647:i32)  [unwired: 1 in, 8 out]
              n239 = Greater Than 0?(x=w647) -> (x > 0?=w651:bool)
            }
            n240 = case shown="False" w638 {
              tunnel: w637 -> [w644 w646]
              tunnel: w635 -> [w643 _]
              tunnel: [w642 w646] -> w634
              tunnel: w633 -> [w639 _]
              tunnel: w632 -> [w641 w645]
              tunnel: [w640 w645] -> w631
              frame False {
                n241 = Build Array (concatenate)(w644, w643) -> (w642:string[])
                n242 = Build Array (concatenate)(w641, w639) -> (w640:i32[])
              }
              frame True {
              }
            }
          }
          n243 = for {
            shift-right: [w669] -> w618
            shift-left: w619 -> [w666]
            shift-right: [w667] -> w617
            shift-left: w619 -> [w668]
            tunnel: w607 -> [w655] mode=indexing
            tunnel: w606 -> [w665] mode=indexing
            tunnel: w614 -> [w654] mode=indexing
            # "Connect to controller and query *IDN?"
            n244 = Bundle By Name(cluster=T2 {"Host address/name"="localhost", "Port"=3000, "Board"=0} ("TCP/IP\nConfiguration"), "Host address/name"=w655, "Port"=w665) -> (w661:T2)
            n245 = Number To Decimal String(number=w665) -> (decimal integer string=w658:string)  [unwired: 1 out]
            n246 = local read "System number"() -> (w652:i32)
            n247 = call "PI Open Interface of one system.vi"("System number"=w652, "Interface configuration"=T4 {"RS232 Portnumber"=0, "Timeout"=1000, "RS232 Baud rate"=57600, "Interface"=3, "GPIB Bus"=0, "GPIB Address"=4, "GPIB Mode"=0}, "String to Send"="*idn?", "TCP/IP\nConfiguration"=w661) -> ("String read"=w657:string, "error out"=w653:errorcluster)  [unwired: 8 in, 6 out]
            n248 = Not Equal?(x=w657, y="") -> (x != y?=w656:bool)
            n249 = case shown="False" w656 {
              tunnel: [w678 w684] -> w659
              tunnel: w658 -> [_ w682]
              tunnel: w657 -> [_ w681]
              tunnel: w655 -> [w671 w679]
              tunnel: w654 -> [w677 _]
              frame False {
                n250 = Search and Replace String(replace all?=TRUE, input string=w677, search string="\u0000", replace string="") -> (result string=w673:string)  [unwired: 1 in, 6 out]
                n251 = Concatenate Strings(w673, " -- already connected to another host" ("string"), " -- at address: " ("string"), w671) -> (w678:string)
              }
              frame True {
                n252 = Concatenate Strings(w681, " -- listening on port " ("string"), w682, " -- at address: " ("string"), w679) -> (w684:string)
              }
            }
            n253 = Build Array (concatenate)(w666, w659) -> (w669:string[])
            n254 = Build Array (concatenate)(w668, w655) -> (w667:string[])
            n255 = call "Close connection if open.vi"("System no."=w652, "error in"=w653) -> ()  [unwired: 1 in, 17 out]
          }
          n256 = Array Size(array=w618) -> (size(s)=w630:i32)
          n257 = Equal To 0?(x=w630) -> (x = 0?=w629:bool)
          n258 = case shown="True" w629 {
            tunnel: [w870 w872] -> w627
            tunnel: w628 -> [w870 w871]
            frame False {
            }
            frame True {
              n259 = Bundle By Name(cluster=w871, "status"=TRUE, "code"=100 ("Bundle Element"), "source"="Controller not found" ("Bundle Element")) -> (w872:errorcluster)
            }
          }
        }
      }
      n260 = flat-sequence {
        tunnel: w19 -> [_]
        frame #0 {
          n261 = local write "stop"(FALSE ("stop")) -> ()
        }
      }
    }
    frame Error {
    }
  }
  "error out" <- w13
  "Address" <- w9
  "ID" <- w8
  "All IDs" <- w2
  "All Addresses" <- w1
